vi "ReadLEDState.vi"(4 "String":string) -> (0 "BLUE":bool, 1 "GREEN":bool, 2 "RED":bool)   [LabVIEW 2016]
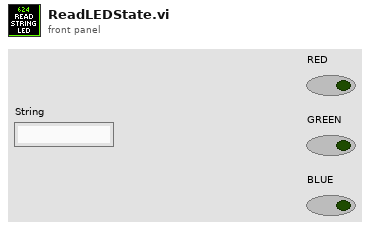
[diagram p1: front panel]
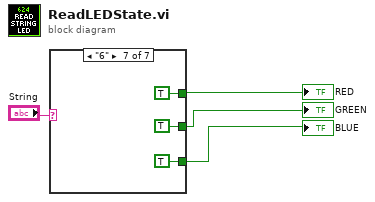
[diagram p0: block diagram]
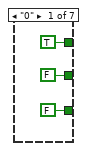
[diagram p2: hidden frame]
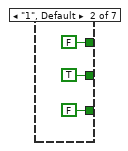
[diagram p3: hidden frame]
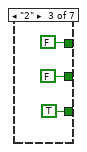
[diagram p4: hidden frame]
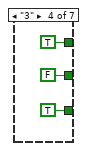
[diagram p5: hidden frame]
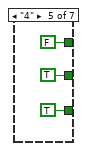
[diagram p6: hidden frame]
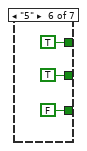
[diagram p7: hidden frame]
diagram:
  n1 = case shown="\"6\"" "String" {
    tunnel: [TRUE FALSE FALSE TRUE FALSE TRUE TRUE] -> w3
    tunnel: [FALSE TRUE FALSE FALSE TRUE TRUE TRUE] -> w2
    tunnel: [FALSE FALSE TRUE TRUE TRUE FALSE TRUE] -> w1
    frame "0" {
    }
    frame "1", Default {
    }
    frame "2" {
    }
    frame "3" {
    }
    frame "4" {
    }
    frame "5" {
    }
    frame "6" {
    }
  }
  "RED" <- w3
  "GREEN" <- w2
  "BLUE" <- w1
